vi "ControlScope.vi"(0 "VISA resource name":refnum<visa-resource-name>, 5 "error in (no error)":errorcluster, 6 "Timebase (1E-6 s)":dbl=1e-06) -> (14 "VISA resource name out":refnum<visa-resource-name>, 15 "Frequency":ext, 16 "Voltage In":ext, 17 "Voltage Out":ext, 19 "error out":errorcluster)   [LabVIEW 2014]
uses:
  <instrlib>/Agilent DSO1000 Series/Agilent DSO1000 Series.lvlib
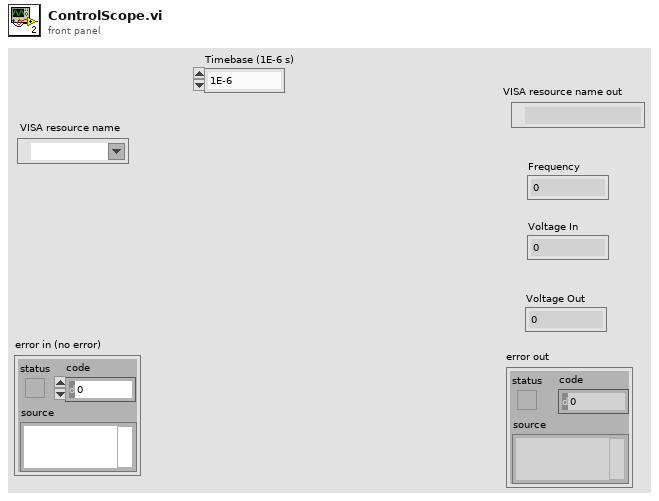
[diagram p1: front panel]
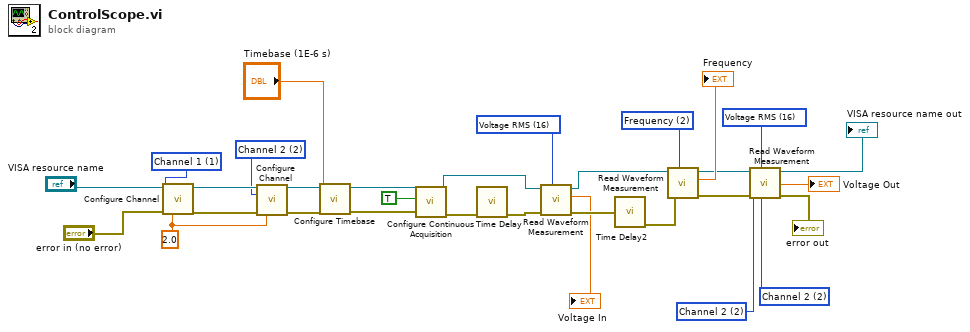
[diagram p0: block diagram]
diagram:
  w1 = u16 2 items=["Channel 1"=1, "Channel 2"=2, "Channel 3"=3, "Channel 4"=4] ("Channel (1: Channel 1)")
  w15 = u16 1 items=["Channel 1"=1, "Channel 2"=2, "Channel 3"=3, "Channel 4"=4] ("Channel (1: Channel 1)")
  w10 = 2.0 ("Vertical Range (10.0 V)")
  w16 = u16 2 items=["Channel 1"=1, "Channel 2"=2, "Channel 3"=3, "Channel 4"=4] ("Source Channel (1: Channel 1)")
  w20 = u16 16 items=["Rise Time", "Fall Time", "Frequency", "Duty Cycle Negative", "Duty Cycle Positive", "Width Negative", "Width Positive", "Over Shoot", "Pre Shoot", "Period", "Amplitude", "Voltage Average", "Voltage Base", "Voltage Max", "Voltage Min", "Voltage Vpp", "Voltage RMS", "Voltage Top", "Phase Negative", "Phase Positive", "Delay Negative", "Delay Positive"] ("Measurement Function (0: Rise Time)")
  w21 = u16 2 items=["Channel 1"=1, "Channel 2"=2, "Channel 3"=3, "Channel 4"=4] ("Source Channel 2 (2: Channel 2)")
  w28 = u16 2 items=["Rise Time", "Fall Time", "Frequency", "Duty Cycle Negative", "Duty Cycle Positive", "Width Negative", "Width Positive", "Over Shoot", "Pre Shoot", "Period", "Amplitude", "Voltage Average", "Voltage Base", "Voltage Max", "Voltage Min", "Voltage Vpp", "Voltage RMS", "Voltage Top", "Phase Negative", "Phase Positive", "Delay Negative", "Delay Positive"] ("Measurement Function (0: Rise Time)")
  w19 = u16 16 items=["Rise Time", "Fall Time", "Frequency", "Duty Cycle Negative", "Duty Cycle Positive", "Width Negative", "Width Positive", "Over Shoot", "Pre Shoot", "Period", "Amplitude", "Voltage Average", "Voltage Base", "Voltage Max", "Voltage Min", "Voltage Vpp", "Voltage RMS", "Voltage Top", "Phase Negative", "Phase Positive", "Delay Negative", "Delay Positive"] ("Measurement Function (0: Rise Time)")
  n1 = call <instrlib>:"Configure Channel.vi"("VISA resource name"="VISA resource name", "Channel (1: Channel 1)"=w15, "error in (no error)"="error in (no error)", "Vertical Range (10.0 V)"=w10) -> ("VISA resource name out"=w11:refnum<visa-resource-name>, "error out"=w13:errorcluster)  [unwired: 10 in]
  n2 = call <instrlib>:"Configure Channel.vi"("VISA resource name"=w11, "Channel (1: Channel 1)"=w1, "error in (no error)"=w13, "Vertical Range (10.0 V)"=w10) -> ("VISA resource name out"=w12:refnum<visa-resource-name>, "error out"=w14:errorcluster)  [unwired: 10 in]
  n3 = call <instrlib>:"Configure Timebase.vi"("error in (no error)"=w14, "Timebase (1E-6 s)"="Timebase (1E-6 s)", "VISA resource name"=w12) -> ("error out"=w7:errorcluster, "VISA resource name out"=w8:refnum<visa-resource-name>)  [unwired: 7 in]
  n4 = call <instrlib>:"Configure Continuous Acquisition.vi"("error in (no error)"=w7, "Enable Continuous Acquisition (T:Enable)"=TRUE, "VISA resource name"=w8) -> ("error out"=w26:errorcluster, "VISA resource name out"=w25:refnum<visa-resource-name>)  [unwired: 7 in]
  n5 = call "Time Delay"("error in (no error)"=w26) -> ("error out"=w31:errorcluster)  [unwired: 10 in]
  n6 = call <instrlib>:"Read Waveform Measurement.vi"("Measurement Function (0: Rise Time)"=w19, "error in (no error)"=w31, "VISA resource name"=w25) -> ("error out"=w30:errorcluster, "Measurement"=→"Voltage In":dbl, "VISA resource name out"=w27:refnum<visa-resource-name>)  [unwired: 6 in]
  n7 = call "Time Delay2"("error in (no error)"=w30) -> ("error out"=w29:errorcluster)  [unwired: 10 in]
  n8 = call <instrlib>:"Read Waveform Measurement.vi"("Measurement Function (0: Rise Time)"=w28, "error in (no error)"=w29, "VISA resource name"=w27) -> ("error out"=w22:errorcluster, "Measurement"=→"Frequency":dbl, "VISA resource name out"=w23:refnum<visa-resource-name>)  [unwired: 6 in]
  n9 = call <instrlib>:"Read Waveform Measurement.vi"("Source Channel 2 (2: Channel 2)"=w21, "Measurement Function (0: Rise Time)"=w20, "error in (no error)"=w22, "Source Channel (1: Channel 1)"=w16, "VISA resource name"=w23) -> ("error out"=→"error out":errorcluster, "Measurement"=→"Voltage Out":dbl, "VISA resource name out"=→"VISA resource name out":refnum<visa-resource-name>)  [unwired: 4 in]
